vi "ActionVIOnDelete.vi"(6 "All deleted Refs":T1[](array[typedef]) format="%.0x", 8 "error in (no error)":errorcluster, 11 "Item Ref in":T1 format="%.0x") -> (0 "error out":errorcluster, 3 "Item Ref out":T1 format="%.0x")   [LabVIEW 2019, in "TimingDRV System Explorer.lvlib"]
uses:
  TimingDRV System Explorer.lvlib
  <vilib>/NI VeriStand/Custom Device API/Custom Device Item Ref.ctl
  NationalInstruments.VeriStand.SystemStorage
  <vilib>/NI Veristand/Custom Device Tools/Custom Device Utility Library/Custom Device Utility Library.lvlib
  <vilib>/NI VeriStand/Custom Device API/Custom Device API.lvlib
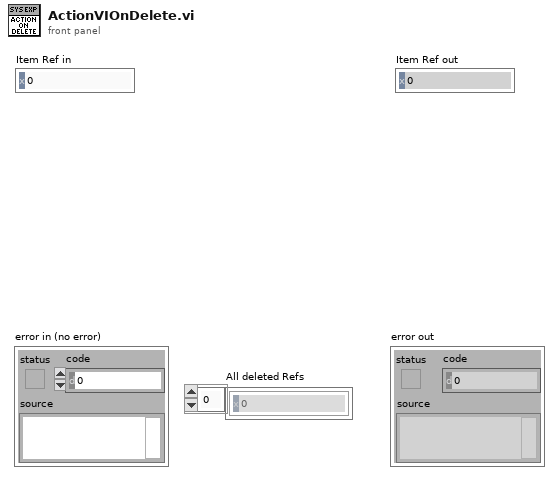
[diagram p1: front panel]
types:
  T1 = typedef "Custom Device API.lvlib/Custom Device Item Ref.ctl" = u64
  T2 = typedef "Custom Device API.lvlib/Custom Device Pointer.ctl" = refnum<k24>
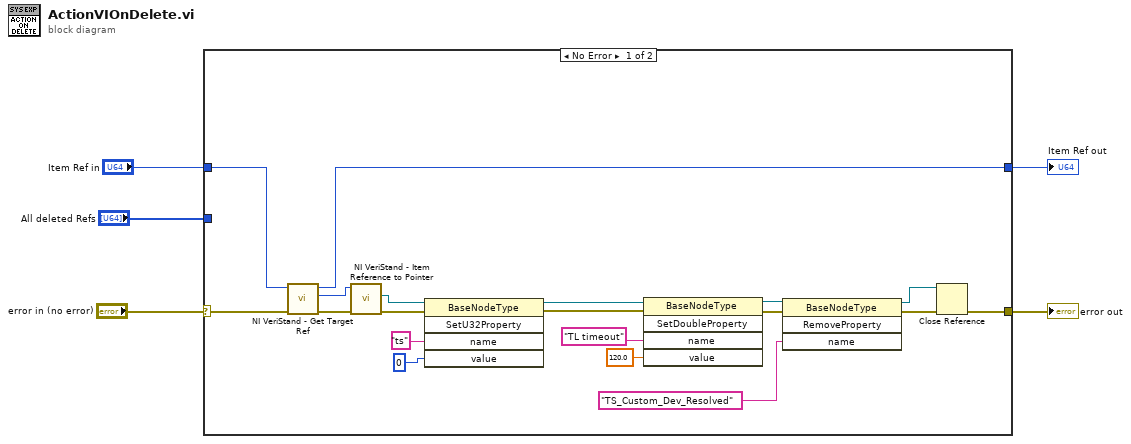
[diagram p0: block diagram]
diagram:
  n1 = case shown="No Error" "error in (no error)" {
    selector: "error in (no error)" -> [w7 w26]
    tunnel: [w6 w26] -> w4
    tunnel: "Item Ref in" -> [w9 w25]
    tunnel: [w8 w25] -> w2
    tunnel: "All deleted Refs" -> [_ _]
    frame No Error {
      n2 = call <vilib>:"NI VeriStand - Get Target Ref.vi"("error in"=w7, "Item Ref in"=w9) -> ("error out"=w24:errorcluster, "Target Ref"=w23:T1, "Item Ref out"=w8:T1)  [unwired: 6 in, 1 out]
      n3 = call <vilib>:"NI VeriStand - Item Reference to Pointer.vi"("error in (no error)"=w24, "Item Ref in"=w23) -> ("error out"=w22:errorcluster, "Node Pointer"=w21:T2)  [unwired: 6 in, 2 out]
      n4 = invoke class="BaseNodeType" method="SetU32Property"(reference=w21, error in=w22, "name"="ts", "value"=u32 0) -> (reference out=w14:T2, error out=w11:errorcluster)  [unwired: 1 in, 3 out]
      n5 = invoke class="BaseNodeType" method="SetDoubleProperty"(reference=w14, error in=w11, "name"="TL timeout", "value"=120.0) -> (reference out=w13:T2, error out=w12:errorcluster)  [unwired: 1 in, 3 out]
      n6 = invoke class="BaseNodeType" method="RemoveProperty"(reference=w13, error in=w12, "name"="TS_Custom_Dev_Resolved") -> (reference out=w17:T2, error out=w16:errorcluster)  [unwired: 1 in, 2 out]
      n7 = Close Reference(reference=w17, error in (no error)=w16) -> (error out=w6:errorcluster)
    }
    frame Error {
    }
  }
  "error out" <- w4
  "Item Ref out" <- w2
